vi "OperadoresConCase.vi"() -> ()   [LabVIEW 2021]
panel:
  out "Resultado":dbl
  in  "Dato B":dbl
  in  "Dato A":dbl
  in  "Decisión":dbl min=0.0 max=4.0
  out "String":string
  in  "stop":bool
  in  "Entrada":bool
  out "Salida negada":bool
  # "Menu de operaciones\n0 - Sin operación\n1 - Suma (A+B)\n2 - Resta (A-B)\n3 - Multiplicación (A*B)\n4 - División (A/B)"
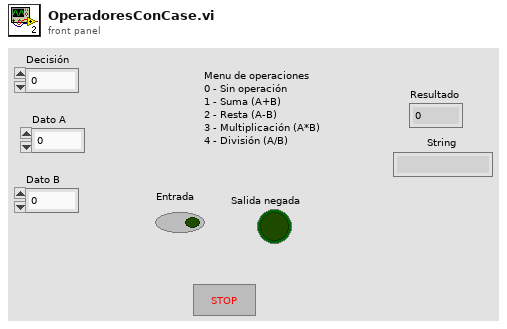
[diagram p1: front panel]
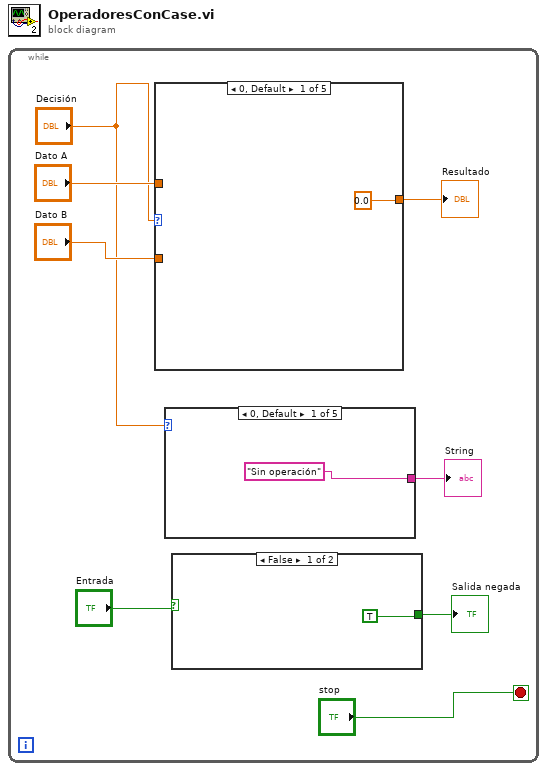
[diagram p0: block diagram]
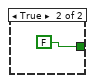
[diagram p2: hidden frame]
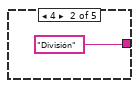
[diagram p3: hidden frame]
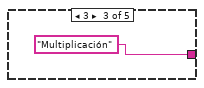
[diagram p4: hidden frame]
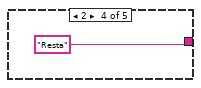
[diagram p5: hidden frame]
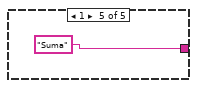
[diagram p6: hidden frame]
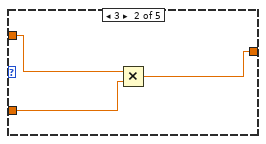
[diagram p7: hidden frame]
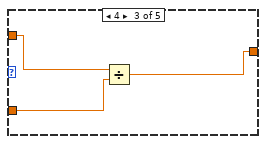
[diagram p8: hidden frame]
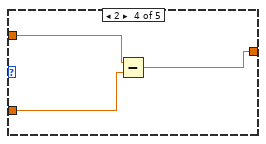
[diagram p9: hidden frame]
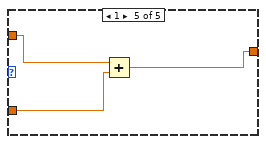
[diagram p10: hidden frame]
diagram:
  n1 = while {
    stop <- "stop" stop-if-true
    n2 = case shown="0, Default" "Decisión" {
      tunnel: "Dato A" -> [_ w19 w21 w25 w28]
      tunnel: "Dato B" -> [_ w18 w22 w24 w27]
      tunnel: [0.0 w17 w20 w23 w26] -> w2
      frame 0, Default {
      }
      frame 3 {
        n3 = Multiply(x=w19, y=w18) -> (x*y=w17:dbl)
      }
      frame 4 {
        n4 = Divide(x=w21, y=w22) -> (x/y=w20:dbl)
      }
      frame 2 {
        n5 = Subtract(x=w25, y=w24) -> (x-y=w23:dbl)
      }
      frame 1 {
        n6 = Add(x=w28, y=w27) -> (x+y=w26:dbl)
      }
    }
    "Resultado" <- w2
    n7 = case shown="0, Default" "Decisión" {
      tunnel: ["Sin operación" "División" "Multiplicación" "Resta" "Suma"] -> w3
      frame 0, Default {
      }
      frame 4 {
      }
      frame 3 {
      }
      frame 2 {
      }
      frame 1 {
      }
    }
    "String" <- w3
    n8 = case shown="False" "Entrada" {
      tunnel: [TRUE FALSE] -> w6
      frame False {
      }
      frame True {
      }
    }
    "Salida negada" <- w6
  }
